vi "Standard ABR.vi"(11 "State (in)":T17) -> (3 "State":T17)   [LabVIEW 2020]
uses:
  epl-vi-lib/Utility VIs/Buttons/KCheckmarkBoolean 2.ctl
  CFTS VIs/CFTS-Experiment State.ctl
  Typedefs/ABR-Analysis State.ctl
  Threshold Estimation VIs/ABR3-Threshold Estimation Result.ctl
  <vilib>/printing/EasyPrintingControls.llb/layout_options.ctl
  <vilib>/printing/EasyPrintingControls.llb/orientation.ctl
  <vilib>/printing/EasyPrintingControls.llb/panel_scaling_for_page.ctl
  <vilib>/printing/EasyPrintingControls.llb/margins.ctl
  <vilib>/printing/EasyPrintingControls.llb/margin_values.ctl
  <vilib>/printing/EasyPrintingControls.llb/measurement_system.ctl
  <vilib>/printing/EasyPrintingControls.llb/printer_options.ctl
  <vilib>/printing/EasyPrintingControls.llb/printing_method.ctl
  <vilib>/printing/EasyPrintingControls.llb/color_or_monochrome.ctl
  <vilib>/printing/EasyPrintingControls.llb/page_header_options.ctl
  <vilib>/printing/EasyPrintingControls.llb/page_headers.ctl
  <vilib>/printing/EasyPrintingControls.llb/page_header_content_options.ctl
  Typedefs/ABR-Queue Data.ctl
  Typedefs/ABR-Parameters.ctl
  Typedefs/ABR-Stimulus.ctl
  Typedefs/ABR-Sequence.ctl
  Typedefs/ABR-Response.ctl
  Threshold Estimation VIs/ABR3-Threshold Estimation Parameters.ctl
  CFTS VIs/CFTS-Options.ctl
  <vilib>/printing/EasyPrintingControls.llb/contents.ctl
  f492785b-1e3c-4081-aebf-1185a71f0bc8.vi
  epl-vi-lib/Utility VIs/File IO VIs/Read Write Anything/Read Anything.vi
  <vilib>/printing/EasyPrinting.llb/Easy Print VI Panel or Documentation (refnum).vi
  epl-vi-lib/Utility VIs/File IO VIs/Configuration File Wrapper VIs/Config-Write Key (string).vi
  <vilib>/Utility/NIReport.llb/NI_ReportGenerationCore.lvlib
panel:
  out "result":T1
  out "Thr":string caption="Threshold (dB SPL)"
  in  "layout options":T2={"orientation (unchanged)"=0, "panel scaling for page (unchanged)"=0, "margins"={"override VI margins (false)"=FALSE, "margins (1.00)"={"top"=1.0, "left"=1.0, "right"=1.0, "bottom"=1.0}, "measurement system (default)"=0}, "printer options"={"destination printer name (current)"="", "printing method (unchanged)"=0, "color or monochrome (unchanged)"=0}, "page header options"={"page headers (unchanged)"=0, "page header content options"={"Include VI Name"=TRUE, "Include VI Path"=TRUE, "Include Last Modification Date"=TRUE, "Include Date Printed"=TRUE, "Include Page Number"=TRUE, "Include VI Icon"=TRUE}}} {"page header options"."page headers (unchanged)" items=["Unchanged", "Include page headers", "Do not include page headers"]; "printer options"."color or monochrome (unchanged)" items=["Unchanged", "Color/grayscale", "Monochrome"]; "printer options"."printing method (unchanged)" items=["Unchanged", "Standard", "PostScript", "Bitmap"]; "panel scaling for page (unchanged)" items=["Unchanged", "No Scaling", "Scale front panel to fit"]; "orientation (unchanged)" items=["Unchanged", "portrait", "landscape"]; "margins"."measurement system (default)" items=["Default", "US", "Metric"]; "margins"."margins (1.00)"."right" format="%.2f"; "margins"."margins (1.00)"."bottom" format="%.2f"; "margins"."margins (1.00)"."top" format="%.2f"; "margins"."margins (1.00)"."left" format="%.2f"}
  out "CM":cluster{dbl[], dbl[]}[](graph) caption="\"CM\""
  out "Neural":cluster{dbl[], dbl[]}[](graph)
  in  "NOTES":string
  out "Analysis":T14
  in  "Response":T16={"Gain"=10000, "Averages"=512, "Window (ms)"=8.5, "Thr Fast Steps"=1.5} {"Thr Fast Steps" format="%.2f"; "Window (ms)" format="%.2f"}
  in  "CAP or ABR":enum16{"CAP", "ABR"}(ring)=enum."ABR" caption="Measure what"
  out "MAX SPL":dbl=113.05999755859375 format="%.2f"
  out "SPL":dbl=35.0
  out "User":string
  out "Run #":u16=14
  out "ID #":u16=1
  in  "Stimulus":T18={"Destination"=1, "Waveform"=enum."TONE PIP", "Frequency (kHz)"=16.0, "Rep rate (/sec)"=30.0, "Alternate Polarity"=FALSE, "Start (dB)"=20, "Stop (dB)"=80, "Step (dB)"=5} {"Rep rate (/sec)" format="%#_8g"; "Frequency (kHz)" format="%.2f"; "Start (dB)" step=5; "Destination" items=["Right ear", "Left ear", "Speaker"]}
  in  "Norm":T19=TRUE caption="Normalize individual traces"
  out "CLICK I-O":cluster{dbl[], dbl[]}[](graph)
  in  "START":bool
  in  "RETURN":bool
  in  "STOP":bool
  out "TONE I-O":cluster{dbl[], dbl[]}[](graph)
  # "Response"
  # "Running Average"
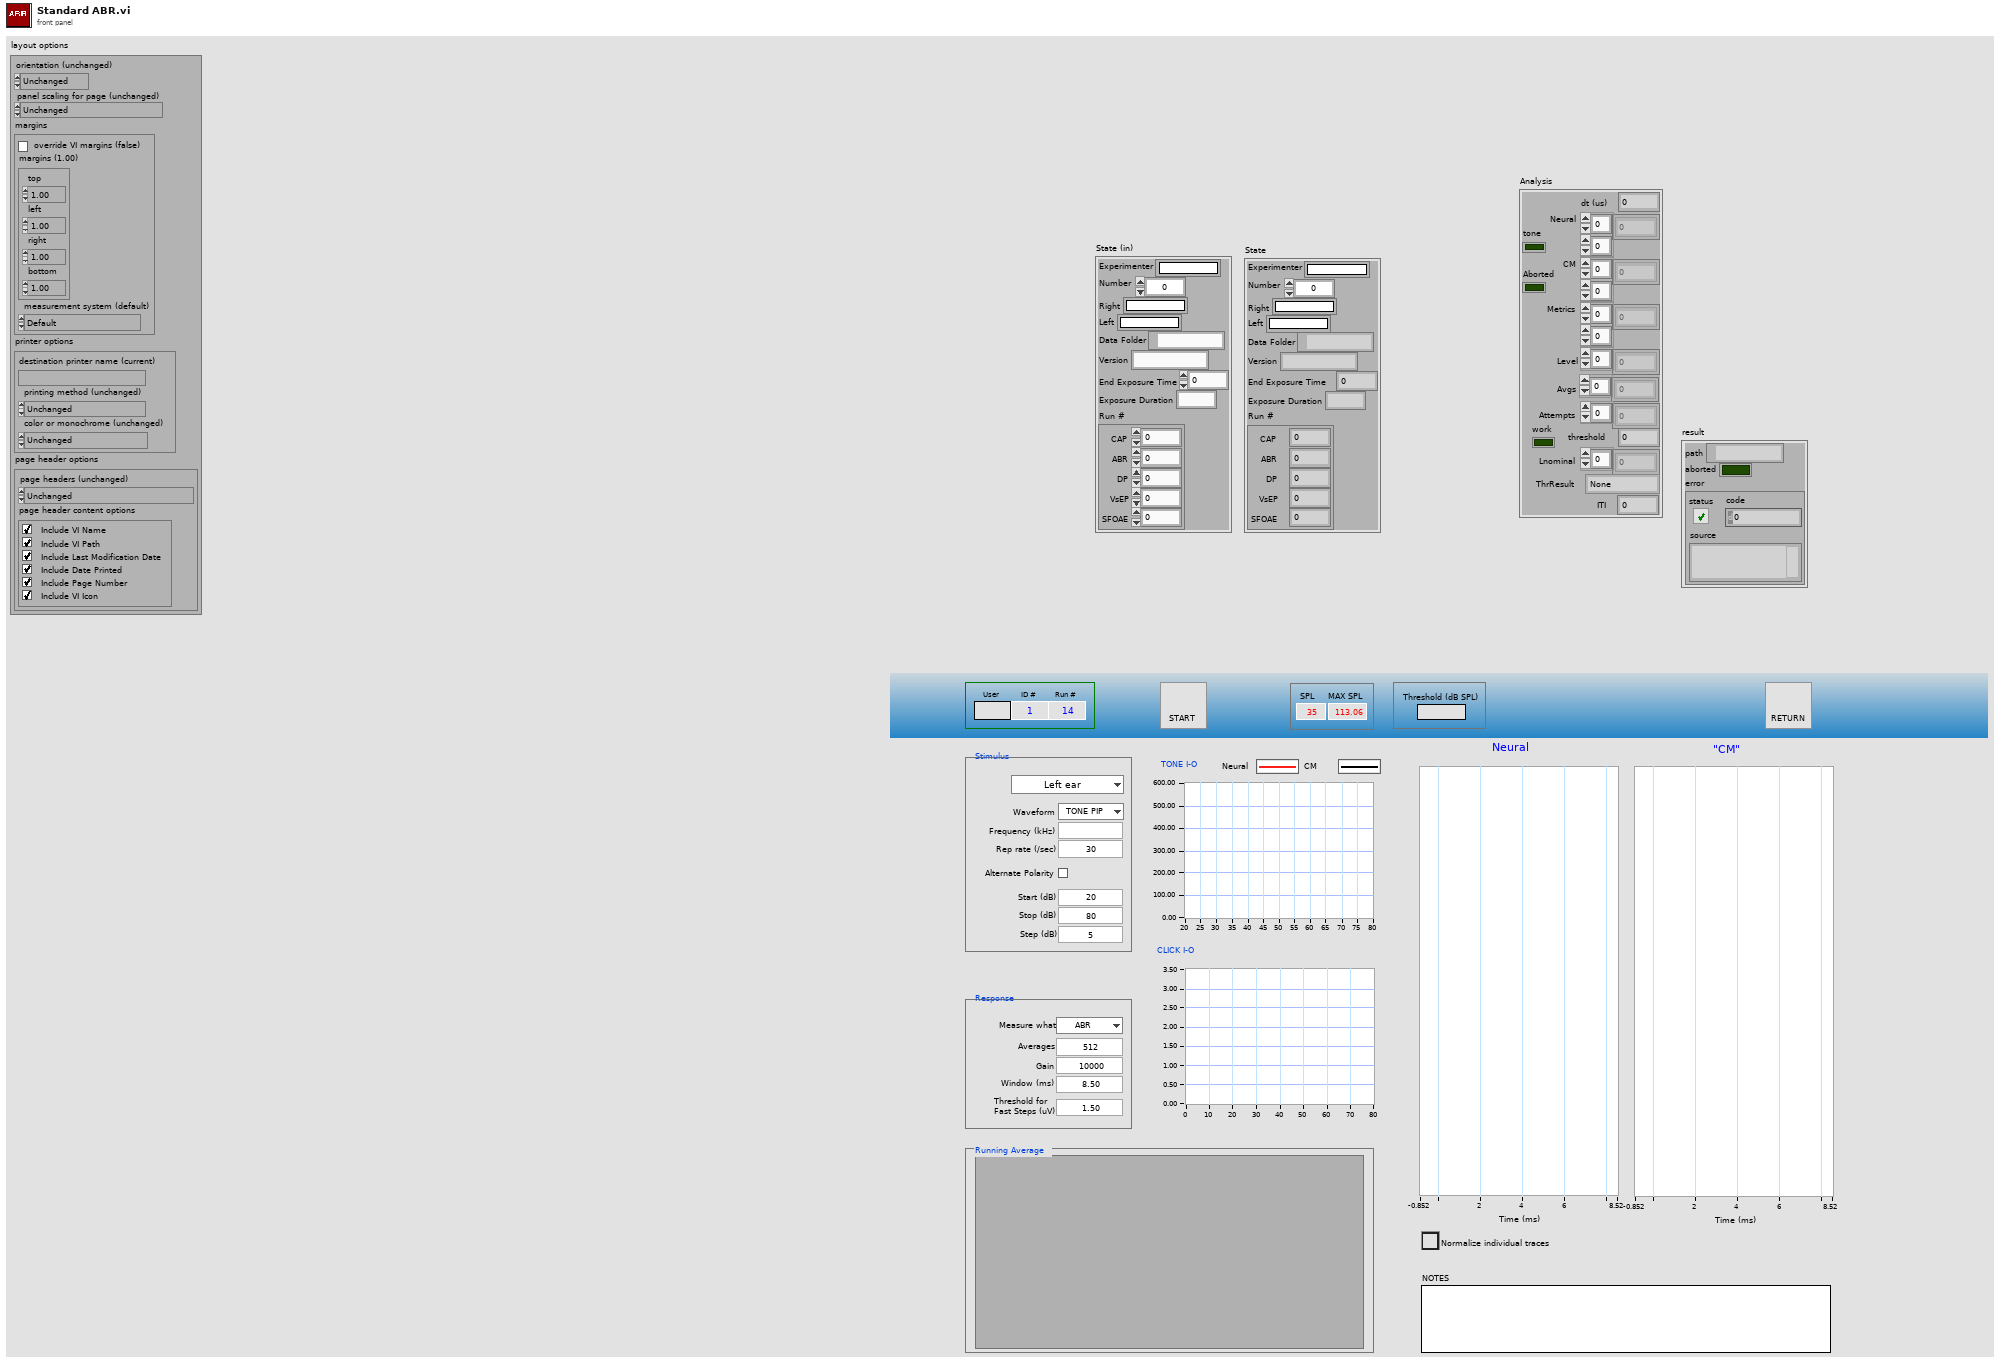
[diagram p1: front panel]
types:
  T1 = cluster{"path":path, "aborted":bool, "error":errorcluster}
  T2 = typedef "NI_ReportGenerationCore.lvlib/layout_options.ctl" = cluster{"orientation (unchanged)":T3, "panel scaling for page (unchanged)":T4, "margins":T5, "printer options":T8, "page header options":T11}
  T3 = typedef "NI_ReportGenerationCore.lvlib/orientation.ctl" = u16
  T4 = typedef "NI_ReportGenerationCore.lvlib/panel_scaling_for_page.ctl" = u16
  T5 = typedef "NI_ReportGenerationCore.lvlib/margins.ctl" = cluster{"override VI margins (false)":bool, "margins (1.00)":T6, "measurement system (default)":T7}
  T6 = typedef "NI_ReportGenerationCore.lvlib/margin_values.ctl" = cluster{"top":dbl, "left":dbl, "right":dbl, "bottom":dbl}
  T7 = typedef "NI_ReportGenerationCore.lvlib/measurement_system.ctl" = u16
  T8 = typedef "NI_ReportGenerationCore.lvlib/printer_options.ctl" = cluster{"destination printer name (current)":string, "printing method (unchanged)":T9, "color or monochrome (unchanged)":T10}
  T9 = typedef "NI_ReportGenerationCore.lvlib/printing_method.ctl" = u16
  T10 = typedef "NI_ReportGenerationCore.lvlib/color_or_monochrome.ctl" = u16
  T11 = typedef "NI_ReportGenerationCore.lvlib/page_header_options.ctl" = cluster{"page headers (unchanged)":T12, "page header content options":T13}
  T12 = typedef "NI_ReportGenerationCore.lvlib/page_headers.ctl" = u16
  T13 = typedef "NI_ReportGenerationCore.lvlib/page_header_content_options.ctl" = cluster{"Include VI Name":bool, "Include VI Path":bool, "Include Last Modification Date":bool, "Include Date Printed":bool, "Include Page Number":bool, "Include VI Icon":bool}
  T14 = typedef "ABR-Analysis State.ctl" = cluster{"dt (us)":dbl, "Neural":dbl[][], "CM":dbl[][], "Metrics":dbl[][], "Level":dbl[], "Avgs":i32[], "Attempts":i32[], "Aborted":bool, "threshold":dbl, "Lnominal":dbl[], "tone":bool, "work":bool, "ThrResult":T15, "ITI":dbl}
  T15 = typedef "ABR3-Threshold Estimation Result.ctl" = enum16{"None", "Power", "Sigmoid", "Power (noisy)", "Suprathreshold", "Invalid"}
  T16 = cluster{"Gain":i32, "Averages":i32, "Window (ms)":sgl, "Thr Fast Steps":sgl}
  T17 = typedef "CFTS-Experiment State.ctl" = cluster{"Experimenter":string, "Number":u32, "Right":string, "Left":string, "Data Folder":path, "Version":string, "End Exposure Time":dbl, "Exposure Duration":string, "Run #":cluster{"CAP":i32, "ABR":i32, "DP":i32, "VsEP":i32, "SFOAE":i32}}
  T18 = cluster{"Destination":u16, "Waveform":enum16{"TONE PIP", "CLICK"}, "Frequency (kHz)":ext, "Rep rate (/sec)":dbl, "Alternate Polarity":bool, "Start (dB)":i32, "Stop (dB)":i32, "Step (dB)":i32}
  T19 = typedef "KCheckmarkBoolean 2.ctl" = bool
  T20 = typedef "ABR-Queue Data.ctl" = cluster{"action":string, "Path":path, "Params":T21, "Threshold Estimation":T25}
  T21 = typedef "ABR-Parameters.ctl" = cluster{"Stimulus":T22, "Sequence":T23, "Response":T24, "Normalize":bool, "Reject":dbl}
  T22 = typedef "ABR-Stimulus.ctl" = cluster{"Destination":string, "Waveform":enum16{"TONE PIP", "CLICK"}, "Frequency (kHz)":ext, "Rep rate (/sec)":dbl, "Alternate Polarity":bool, "Sampling rate (Hz)":dbl, "Duration (ms)":dbl, "Ramp (ms)":dbl, "Click width (us)":dbl, "ITI":enum16{"Rate", "Interval"}}
  T23 = typedef "ABR-Sequence.ctl" = cluster{"Start (dB)":i32, "Stop (dB)":i32, "Step (dB)":i32}
  T24 = typedef "ABR-Response.ctl" = cluster{"CAP or ABR":enum16{"CAP", "ABR"}, "Gain":i32, "Averages":i32, "Window (ms)":sgl, "Thr Fast Steps":sgl, "Fs (Hz)":dbl, "Save raw":bool}
  T25 = typedef "ABR3-Threshold Estimation Parameters.ctl" = cluster{"Tmin (ms)":dbl, "Tmax (ms)":dbl, "CC criterion":dbl, "adjR2 criterion":dbl}
  T26 = cluster{"TONE I-O":refnum<vi>, "Neural":refnum<vi>, "CM":refnum<vi>, "CLICK I-O":refnum<vi>}
  T27 = typedef "ABR-Runtime Data.ctl" = cluster{"Ceiling":dbl, "Threshold":dbl, "Crossed?":bool, "Step":dbl, "Stop":i32, "Avgs":i32, "Level":dbl, "AI Npts":i32, "Doubled?":bool, "dt":dbl, "gain":dbl, "rep pairs/buffer":i32, "NWinPts":i32, "Save raw":bool, "SigMan":refnum<class "SignalManager.lvclass">, "path":path}
  T28 = typedef "ABR-Averaging Result.ctl" = cluster{"navg":i32, "natt":i32, "Neural":dbl[], "Microphonic":dbl[]}
  T29 = cluster{"Datafile path":path, "abort":bool, "error out":errorcluster}
  T30 = typedef "CFTS-Options.ctl" = cluster{"Rig ID":string, "Acoustic System IDs":cluster{"Right":string, "Left":string}, "Extension":string, "Advanced users":string[], "All advanced":bool, "Run vitals":bool, "hash":string, "Allow nonEPL":bool, "NonEPL":string[], "Data root":path}
  T31 = enum8{"Enabled", "Disabled", "Disabled and Grayed Out"}
  T32 = cluster{string, "appended path":path, "Params":T21, "Threshold Estimation":T25}
  T33 = typedef "NI_ReportGenerationCore.lvlib/contents.ctl" = u16
  T34 = typedef "ABR3-Threshold Estimation Work.ctl" = cluster{"Threshold":dbl, "Criterion":dbl, "graphs":cluster{"X":dbl[], "Y":dbl[]}[], "Power2":string, "Sigmoid":string, "Result":T15}
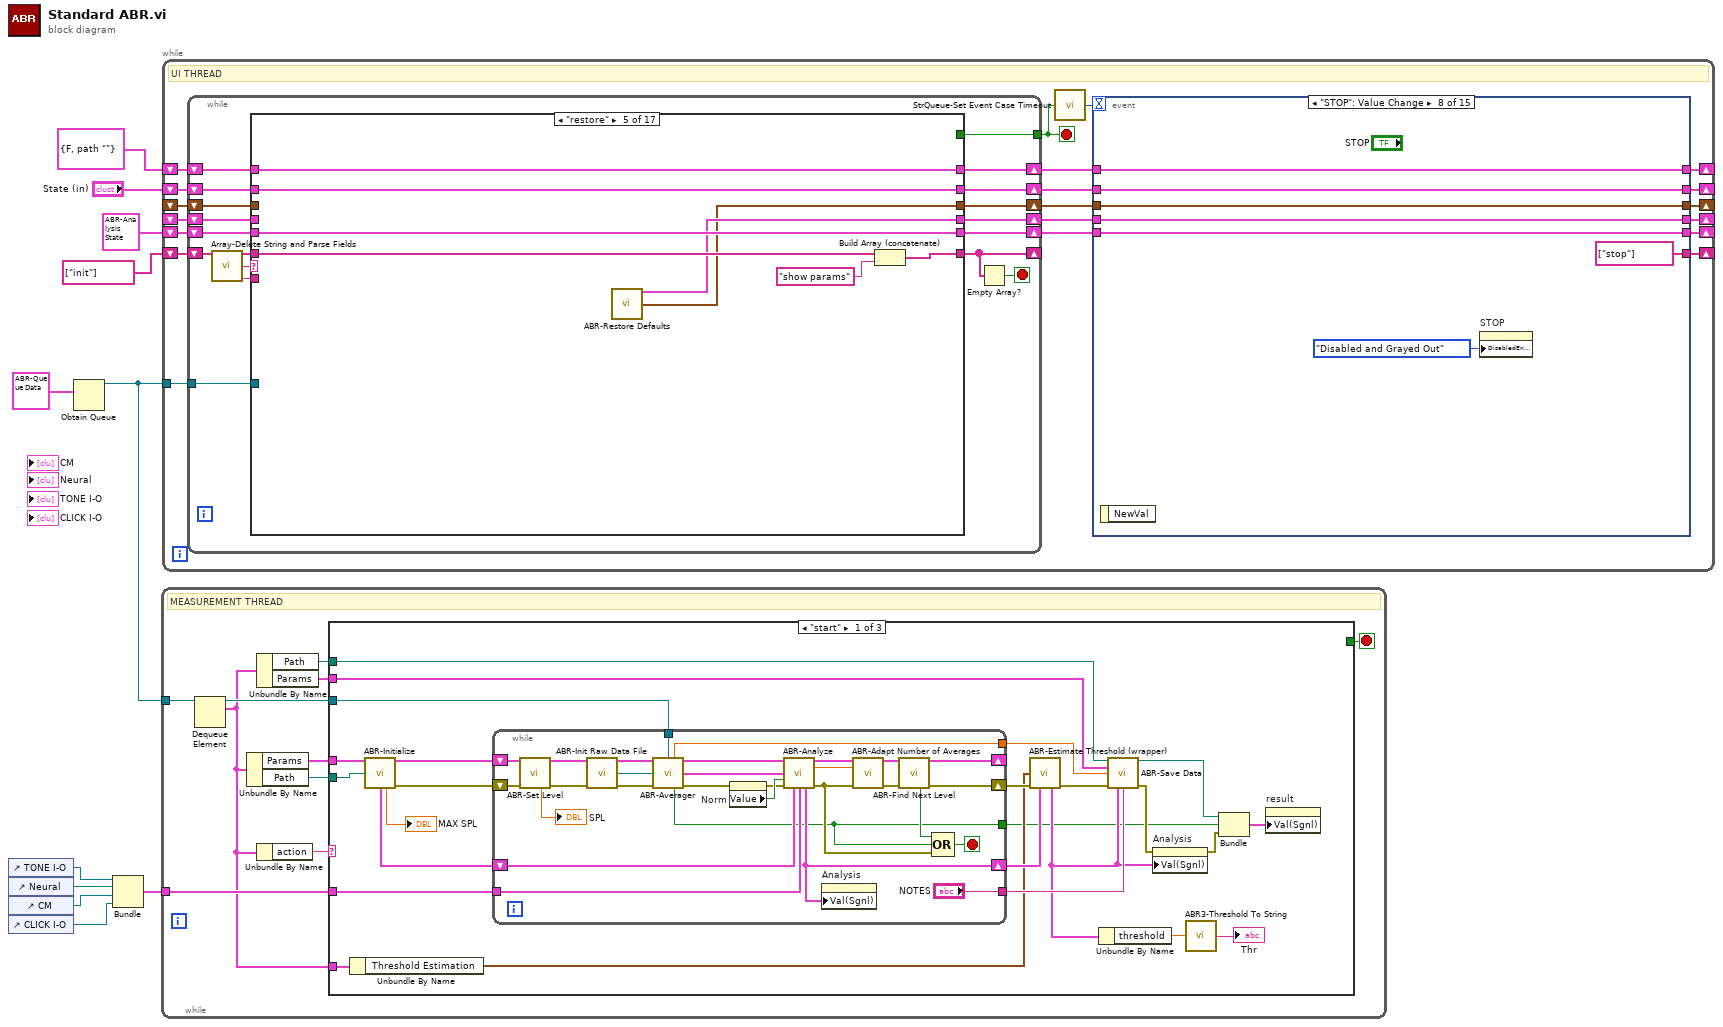
[diagram p0: block diagram]
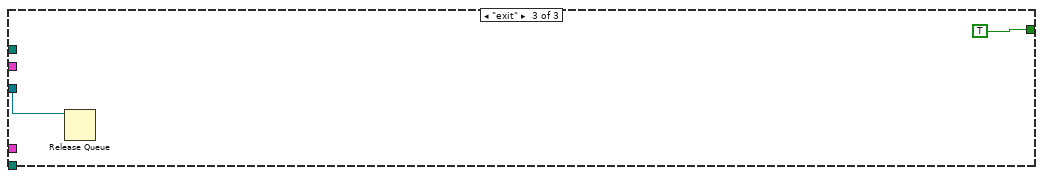
[diagram p3: hidden frame]
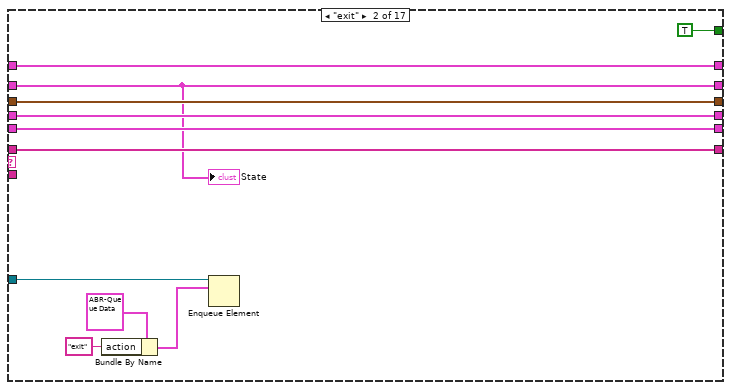
[diagram p5: hidden frame]
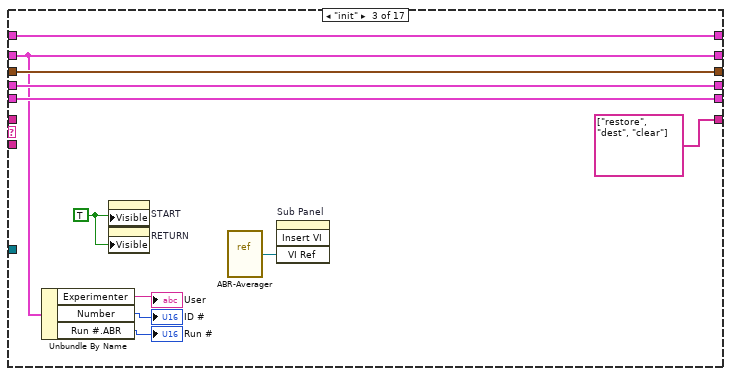
[diagram p6: hidden frame]
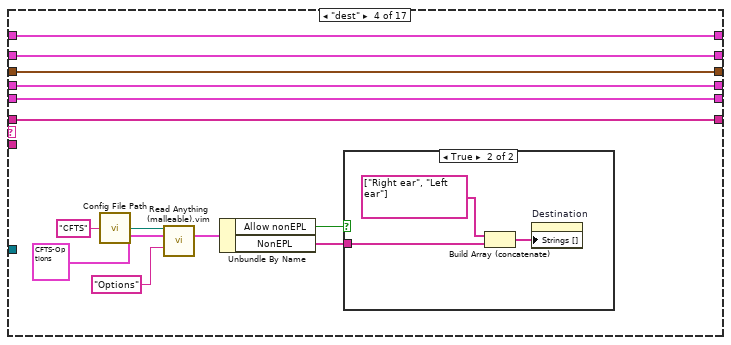
[diagram p7: hidden frame]
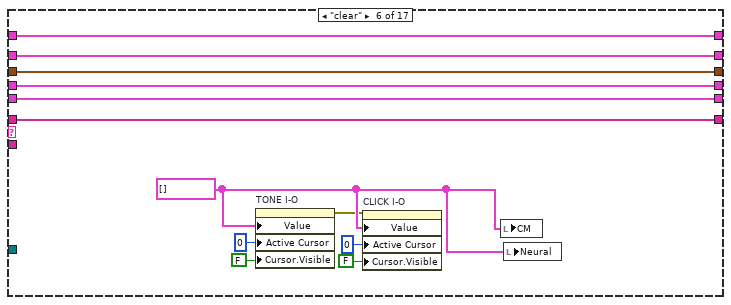
[diagram p9: hidden frame]
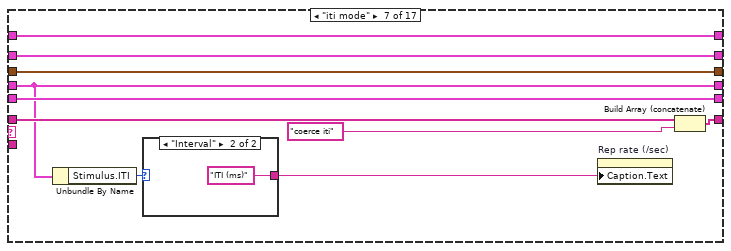
[diagram p10: hidden frame]
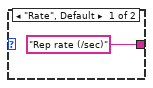
[diagram p11: hidden frame]
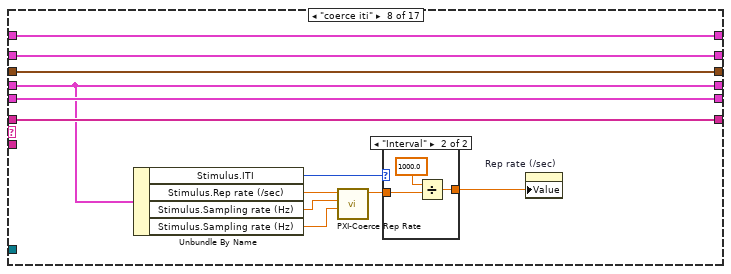
[diagram p12: hidden frame]
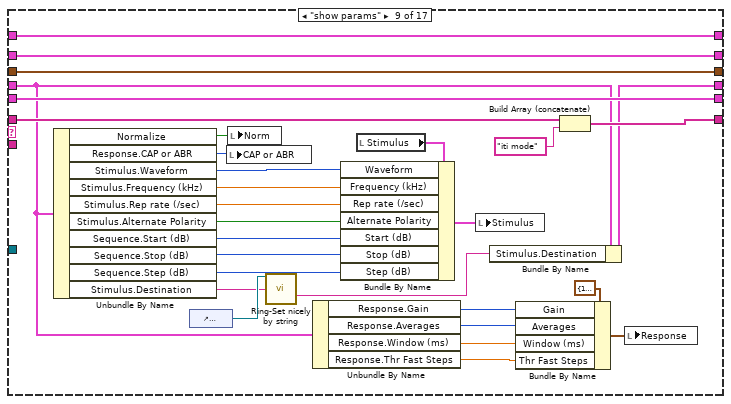
[diagram p14: hidden frame]
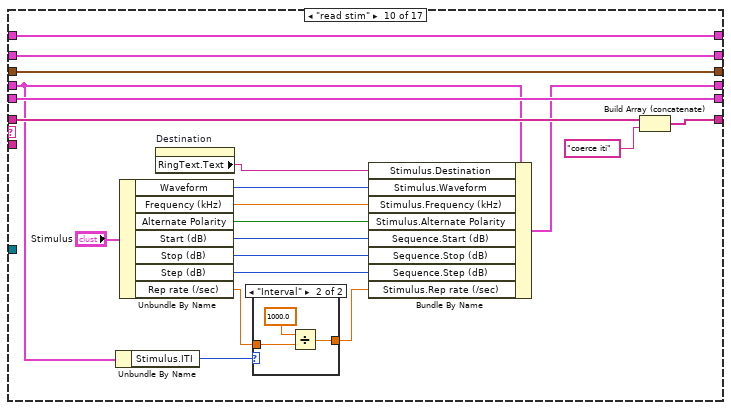
[diagram p15: hidden frame]
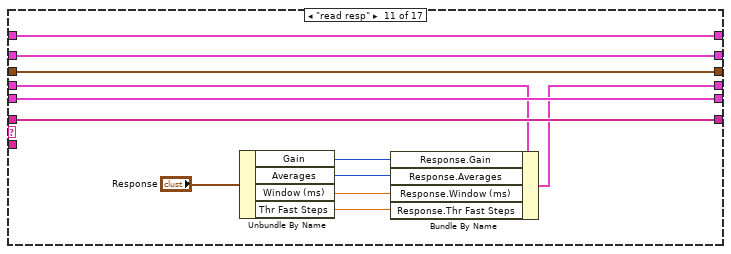
[diagram p17: hidden frame]
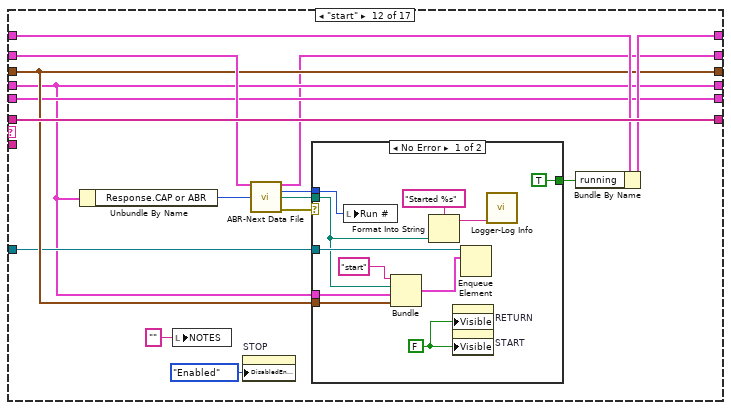
[diagram p18: hidden frame]
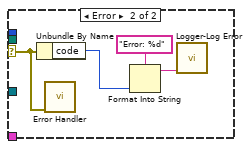
[diagram p19: hidden frame]
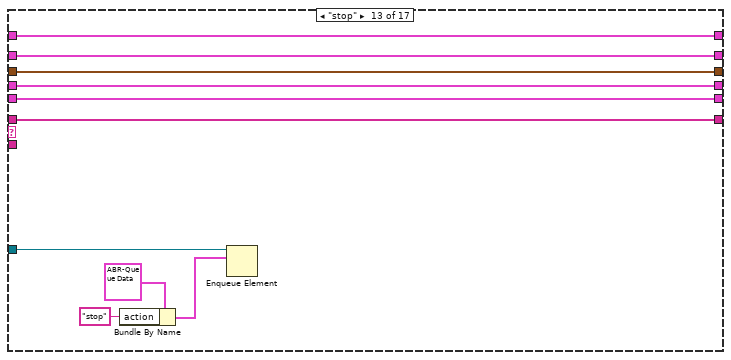
[diagram p20: hidden frame]
diagram:
  n1 = control-ref of="TONE I-O"() -> (w5:refnum<vi>)
  n2 = control-ref of="Neural"() -> (w7:refnum<vi>)
  n3 = control-ref of="CM"() -> (w6:refnum<vi>)
  n4 = control-ref of="CLICK I-O"() -> (w4:refnum<vi>)
  n5 = Obtain Queue(element data type=T20 {"action"="", "Path"=path "", "Params"={"Stimulus"={"Destination"="", "Waveform"=enum."TONE PIP", "Frequency (kHz)"=16.0, "Rep rate (/sec)"=30.0, "Alternate Polarity"=FALSE, "Sampling rate (Hz)"=0.0, "Duration (ms)"=30.0, "Ramp (ms)"=5.0, "Click width (us)"=0.0, "ITI"=enum."Rate"}, "Sequence"={"Start (dB)"=20, "Stop (dB)"=80, "Step (dB)"=5}, "Response"={"CAP or ABR"=enum."ABR", "Gain"=10000, "Averages"=512, "Window (ms)"=8.5, "Thr Fast Steps"=8.5, "Fs (Hz)"=25000.0, "Save raw"=FALSE}, "Normalize"=FALSE, "Reject"=0.0}, "Threshold Estimation"={"Tmin (ms)"=0.0, "Tmax (ms)"=0.0, "CC criterion"=0.0, "adjR2 criterion"=0.0}} ("Cluster")) -> (queue out=w11:refnum<queue>)  [unwired: 4 in, 2 out]
  n6 = Bundle("TONE I-O"=w5, "Neural"=w7, "CM"=w6, "CLICK I-O"=w4) -> (w8:T26)  [unwired: 1 in]
  n7 = while {
    tunnel: w11 -> [w21]
    tunnel: w8 -> [w20]
    stop <- w17 stop-if-true
    # "MEASUREMENT THREAD"
    n8 = Dequeue Element(queue=w21) -> (queue out=w19:refnum<queue>, element=w14:T20)  [unwired: 2 in, 2 out]
    n9 = Unbundle By Name(w14) -> ("Params"=w16:T21, "Path"=w15:path)
    n10 = Unbundle By Name(w14) -> ("Path"=w13:path, "Params"=w12:T21)
    n11 = Unbundle By Name(w14) -> ("action"=w18:string)
    n12 = case shown="\"start\"" w18 {
      tunnel: w20 -> [w46 _ _]
      tunnel: w19 -> [w36 _ w77]
      tunnel: [_ _ TRUE] -> w17
      tunnel: w16 -> [w44 _ _]
      tunnel: w15 -> [w40 _ _]
      tunnel: w14 -> [w31 _ _]
      tunnel: w13 -> [w28 _ _]
      tunnel: w12 -> [w27 _ _]
      frame "start" {
        n13 = Unbundle By Name(w31) -> ("Threshold Estimation"=w30:T25)
        n14 = call "ABR-Initialize.vi"("Params"=w44, "Data path"=w40) -> ("Runtime"=w41:T27, "Analysis"=w42:T14, "Ceiling"=→"MAX SPL":dbl, "error out"=w43:errorcluster)  [unwired: 10 in]
        n15 = while {
          shift-right: [w74] -> w38
          shift-left: w43 -> [w72]
          shift-right: [w70] -> _
          shift-left: w41 -> [w69]
          shift-right: [w60] -> w37
          shift-left: w42 -> [w65]
          tunnel: w46 -> [w64]
          tunnel: ["NOTES"] -> w39
          tunnel: [w51] -> w26
          tunnel: w36 -> [w50]
          tunnel: [w47] -> w22
          stop <- w75 stop-if-true
          # "stepsize"
          # "max SPL"
          # "array of levels"
          # "current SPL"
          n16 = call "ABR-Set Level.vi"("Runtime"=w69, "error in (no error)"=w72) -> ("Runtime thru"=w59:T27, "Level"=→"SPL":dbl, "error out"=w57:errorcluster)  [unwired: 11 in]
          n17 = call "ABR-Init Raw Data File.vi"("Runtime in"=w59, "error in (no error)"=w57) -> ("Runtime out"=w58:T27, "refnum out"=w55:refnum<file>, "error out"=w56:errorcluster)  [unwired: 11 in]
          n18 = call "ABR-Averager.vi"("Runtime"=w58, "queue"=w50, "raw data file"=w55, "error in (no error)"=w56) -> ("Rej Thresh out"=w47:dbl, "Runtime thru"=w54:T27, "result"=w49:T28, "abort"=w51:bool, "error out"=w68:errorcluster)  [unwired: 7 in]
          n19 = property on="Norm" class="Bool (strict)"(error in=w68) -> (error out=w66:errorcluster, "Value"=w67:T19)  [unwired: 1 in, 1 out]
          n20 = call "ABR-Analyze.vi"("Runtime"=w54, "result"=w49, "Normalize individual?"=w67, "error in"=w66, "Analysis in"=w65, "Graphs"=w64) -> ("Runtime thru"=w53:T27, "spread value"=w48:dbl, "Analysis out"=w60:T14, "error out"=w52:errorcluster)  [unwired: 6 in]
          n21 = property on="Analysis" class="Clust (strict)"("Val(Sgnl)"=w60) -> ()  [unwired: 2 in, 2 out]
          n22 = call "ABR-Adapt Number of Averages.vi"("Runtime"=w53, "Amplitude"=w48, "error in (no error)"=w52) -> ("Runtime out"=w63:T27, "error out"=w62:errorcluster)  [unwired: 11 in]
          n23 = call "ABR-Find Next Level.vi"("Runtime"=w63, "error in (no error)"=w62) -> ("Runtime out"=w70:T27, "Finished"=w73:bool, "error out"=w74:errorcluster)  [unwired: 11 in]
          n24 = Compound Arithmetic op=OR(w73, w51, w52) -> (w75:bool)
        }
        n25 = call "ABR-Estimate Threshold (wrapper).vi"("Threshold Estimation"=w30, "error in (no error)"=w38, "Analysis (in)"=w37) -> ("Analysis (out)"=w32:T14, "error out"=w35:errorcluster)  [unwired: 10 in, 1 out]
        n26 = Unbundle By Name(w32) -> ("threshold"=w33:dbl)
        n27 = call "ABR-Save Data.vi"("file path"=w28, "Params"=w27, "reject"=w22, "error in (no error)"=w35, "Analysis"=w32, "Notes"=w39) -> ("Datafile path"=w24:path, "error out"=w29:errorcluster)  [unwired: 8 in]
        n28 = property on="Analysis" class="Clust (strict)"(error in=w29, "Val(Sgnl)"=w32) -> (error out=w25:errorcluster)  [unwired: 1 in, 1 out]
        n29 = call "ABR3-Threshold To String.vi"("Threshold"=w33) -> ("String"=→"Thr":string)
        n30 = Bundle("Datafile path"=w24, "abort"=w26, "error out"=w25) -> (w23:T29)  [unwired: 1 in]
        n31 = property on="result" class="Clust (strict)"("Val(Sgnl)"=w23) -> ()  [unwired: 2 in, 2 out]
      }
      frame "stop", Default {
      }
      frame "exit" {
        n32 = Release Queue(queue=w77) -> ()  [unwired: 2 in, 3 out]
      }
    }
  }
  n33 = while {
    tunnel: w11 -> [w83]
    shift-right: [w90] -> _
    shift-left: _ -> [w88]
    shift-right: [w91] -> _
    shift-left: T14 {"dt (us)"=0.0, "Neural"=[], "CM"=[], "Metrics"=[], "Level"=[], "Avgs"=[], "Attempts"=[], "Aborted"=FALSE, "threshold"=0.0, "Lnominal"=[], "tone"=FALSE, "work"=FALSE, "ThrResult"=enum."None", "ITI"=0.0} ("Analysis") -> [w92]
    shift-right: [w89] -> _
    shift-left: _ -> [w86]
    shift-right: [w96] -> _
    shift-left: string[] ["init"] -> [w97]
    shift-right: [w80] -> _
    shift-left: cluster{"running":bool, "path":path} {"running"=FALSE, "path"=path ""} -> [w82]
    shift-right: [w79] -> _
    shift-left: "State (in)" -> [w84]
    stop <- w94 stop-if-true
    # "UI THREAD"
    n34 = while {
      shift-right: [w114] -> _
      shift-left: w97 -> [w100]
      tunnel: [w112] -> w94
      shift-right: [w109] -> w85
      shift-left: w88 -> [w108]
      shift-right: [w111] -> w93
      shift-left: w92 -> [w110]
      shift-right: [w107] -> w87
      shift-left: w86 -> [w106]
      tunnel: w83 -> [w104]
      shift-right: [w102] -> w81
      shift-left: w82 -> [w103]
      shift-right: [w101] -> w78
      shift-left: w84 -> [w105]
      stop <- w113 stop-if-true
      n35 = call "Array-Delete String and Parse Fields.vi"("Array in"=w100) -> ("Array out"=w115:string[], "Field 1"=w99:string, "Field 2"=w98:string)  [unwired: 10 in, 2 out]
      n36 = case shown="\"restore\"" w99 {
        tunnel: w115 -> [w121 w132 _ w156 w167 w179 w189 w203 w236 w256 w272 w288 w313 w323 w362 w378 w392]
        tunnel: [w121 w132 string[] ["restore", "dest", "clear"] w156 w161 w179 w187 w203 w235 w255 w272 w288 w313 w321 w362 w378 w392] -> w114
        tunnel: [_ TRUE _ _ _ _ _ _ _ _ _ _ _ _ _ _ _] -> w112
        tunnel: [w118 w130 w143 w155 w166 w178 w184 w201 w233 w253 w270 w282 w312 w328 w355 w363 w383] -> w111
        tunnel: w110 -> [w118 w130 w143 w155 w166 w178 w184 w201 w233 w253 w270 w282 w312 w328 w355 w363 w384]
        tunnel: [w119 w129 w142 w154 w165 w177 w183 w195 w212 w242 w261 w280 w311 w314 w361 w377 w391] -> w109
        tunnel: w108 -> [w119 w129 w142 w154 _ w177 w183 w195 w214 w240 w266 w280 w311 w314 w361 w377 w391]
        tunnel: [w120 w128 w141 w153 w164 w176 w185 w202 w234 w254 w271 w283 w310 w327 w360 w376 w385] -> w107
        tunnel: w106 -> [w120 w128 w141 w153 _ w176 w185 w202 w234 w254 w271 w283 w310 w327 w360 w376 w385]
        tunnel: w105 -> [w116 w122 w137 w151 w162 w168 w180 w199 w209 w244 w268 w284 w308 w318 w358 w374 w382]
        tunnel: w104 -> [_ w125 _ _ _ _ _ _ _ _ _ w281 w304 _ _ _ _]
        tunnel: w103 -> [w117 w123 w133 w152 w163 w169 w181 w200 w210 w245 w269 w287 w309 w317 w359 w375 w390]
        tunnel: [w117 w123 w133 w152 w163 w169 w181 w200 w210 w245 w269 w285 w309 w316 w359 w375 w390] -> w102
        tunnel: [w116 w122 w137 w151 w162 w168 w180 w199 w209 w244 w268 w273 w308 w315 w358 w374 w382] -> w101
        tunnel: w98 -> [_ _ _ _ _ _ _ _ _ _ _ _ _ w320 _ _ _]
        frame "", Default {
        }
        frame "exit" {
          n37 = Bundle By Name(cluster=T20 {"action"="", "Path"=path "", "Params"={"Stimulus"={"Destination"="", "Waveform"=enum."TONE PIP", "Frequency (kHz)"=16.0, "Rep rate (/sec)"=30.0, "Alternate Polarity"=FALSE, "Sampling rate (Hz)"=0.0, "Duration (ms)"=30.0, "Ramp (ms)"=5.0, "Click width (us)"=0.0, "ITI"=enum."Rate"}, "Sequence"={"Start (dB)"=20, "Stop (dB)"=80, "Step (dB)"=5}, "Response"={"CAP or ABR"=enum."ABR", "Gain"=10000, "Averages"=512, "Window (ms)"=8.5, "Thr Fast Steps"=8.5, "Fs (Hz)"=25000.0, "Save raw"=FALSE}, "Normalize"=FALSE, "Reject"=0.0}, "Threshold Estimation"={"Tmin (ms)"=0.0, "Tmax (ms)"=0.0, "CC criterion"=0.0, "adjR2 criterion"=0.0}} ("Cluster"), "action"="exit") -> (w124:T20)
          n38 = Enqueue Element(queue=w125, element=w124) -> ()  [unwired: 2 in, 3 out]
          "State" <- w122
        }
        frame "init" {
          w136 = TRUE
          n39 = Unbundle By Name(w137) -> ("Experimenter"=→"User":string, "Number"=→"ID #":u32, "Run #.ABR"=→"Run #":i32)
          n40 = property on="START" class="Bool"("Visible"=w136) -> ()  [unwired: 2 in, 2 out]
          n41 = property on="RETURN" class="Bool"("Visible"=w136) -> ()  [unwired: 2 in, 2 out]
          n42 = vi-ref "ABR-Averager.vi"() -> (w135:refnum<vi>)
          n43 = invoke on="Sub Panel" class="SubPanel" method="Insert VI"("VI Ref"=w135) -> ()  [unwired: 3 in, 4 out]
        }
        frame "dest" {
          n44 = call "Config File Path.vi"("AppName"="CFTS") -> ("Default config file name"=w149:path)
          n45 = call "Read Anything (malleable).vim"("Config file path"=w149, "Options in"=T30 {"Rig ID"="", "Acoustic System IDs"={"Right"="", "Left"=""}, "Extension"="", "Advanced users"=[], "All advanced"=FALSE, "Run vitals"=FALSE, "hash"="", "Allow nonEPL"=FALSE, "NonEPL"=[], "Data root"=path ""} ("Options"), "Section"="Options") -> ("Options out"=w146:T30)  [unwired: 9 in, 3 out]
          n46 = Unbundle By Name(w146) -> ("Allow nonEPL"=w145:bool, "NonEPL"=w144:string[])
          n47 = case shown="True" w145 {
            tunnel: w144 -> [_ w159]
            frame False {
            }
            frame True {
              n48 = Build Array (concatenate)(string[] ["Right ear", "Left ear"], w159) -> (w157:string[])
              n49 = property on="Destination" class="Ring (strict)"("Strings []"=w157) -> ()  [unwired: 2 in, 2 out]
            }
          }
        }
        frame "restore" {
          n50 = call "ABR-Restore Defaults.vi"() -> ("Params"=w165:T21, "Threshold Estimation"=w164:T25)  [unwired: 13 in, 1 out]
          n51 = Build Array (concatenate)(w167, "show params") -> (w161:string[])
        }
        frame "clear" {
          w175 = cluster{dbl[], dbl[]}[] [] ("TONE I-O")
          n52 = property on="TONE I-O" class="XYGraph (strict)"("Value"=w175, "Active Cursor"=u32 0, "Cursor.Visible"=FALSE) -> (error out=w172:errorcluster)  [unwired: 2 in, 1 out]
          n53 = property on="CLICK I-O" class="XYGraph (strict)"(error in=w172, "Value"=w175, "Active Cursor"=u32 0, "Cursor.Visible"=FALSE) -> ()  [unwired: 1 in, 2 out]
          n54 = local write "CM"(w175) -> ()
          n55 = local write "Neural"(w175) -> ()
        }
        frame "iti mode" {
          n56 = Unbundle By Name(w183) -> ("Stimulus.ITI"=w182:enum16{"Rate", "Interval"})
          n57 = case shown="\"Interval\"" w182 {
            tunnel: ["Rep rate (/sec)" ("Caption.Text") "ITI (ms)" ("Caption.Text")] -> w188
            frame "Rate", Default {
            }
            frame "Interval" {
            }
          }
          n58 = property on="Rep rate (/sec)" class="DigNum (strict)"("Caption.Text"=w188) -> ()  [unwired: 2 in, 2 out]
          n59 = Build Array (concatenate)(w189, "coerce iti") -> (w187:string[])
        }
        frame "coerce iti" {
          n60 = Unbundle By Name(w195) -> ("Stimulus.ITI"=w192:enum16{"Rate", "Interval"}, "Stimulus.Rep rate (/sec)"=w196:dbl, "Stimulus.Sampling rate (Hz)"=w194:dbl, "Stimulus.Sampling rate (Hz)"=w193:dbl)
          n61 = call "PXI-Coerce Rep Rate.vi"("AI sampling rate (Hz)"=w193, "AO sampling rate (Hz)"=w194, "Rep rate (Hz)"=w196) -> ("Coerced rep rate (Hz)"=w198:dbl)  [unwired: 5 in, 3 out]
          n62 = case shown="\"Interval\"" w192 {
            tunnel: w198 -> [w204 w207]
            tunnel: [w204 w206] -> w197
            frame "Rate", Default {
            }
            frame "Interval" {
              n63 = Divide(x=1000.0, y=w207) -> (x/y=w206:dbl)
            }
          }
          n64 = property on="Rep rate (/sec)" class="DigNum (strict)"("Value"=w197) -> ()  [unwired: 2 in, 2 out]
        }
        frame "show params" {
          n65 = Unbundle By Name(w214) -> ("Normalize"=w208:bool, "Response.CAP or ABR"=w232:enum16{"CAP", "ABR"}, "Stimulus.Waveform"=w230:enum16{"TONE PIP", "CLICK"}, "Stimulus.Frequency (kHz)"=w229:ext, "Stimulus.Rep rate (/sec)"=w228:dbl, "Stimulus.Alternate Polarity"=w227:bool, "Sequence.Start (dB)"=w226:i32, "Sequence.Stop (dB)"=w225:i32, "Sequence.Step (dB)"=w224:i32, "Stimulus.Destination"=w221:string)
          n66 = control-ref of="Destination"() -> (w222:refnum<vi>)
          n67 = local write "CAP or ABR"(w232) -> ()
          n68 = local write "Norm"(w208) -> ()
          n69 = call "Ring-Set nicely by string.vi"("Ring in"=w222, "Device"=w221) -> ("Selection"=w211:string)  [unwired: 9 in, 4 out]
          n70 = Unbundle By Name(w214) -> ("Response.Gain"=w220:i32, "Response.Averages"=w219:i32, "Response.Window (ms)"=w218:sgl, "Response.Thr Fast Steps"=w217:sgl)
          n71 = local read "Stimulus"() -> (w231:T18)
          n72 = Bundle By Name(cluster=w231, "Waveform"=w230, "Frequency (kHz)"=w229, "Rep rate (/sec)"=w228, "Alternate Polarity"=w227, "Start (dB)"=w226, "Stop (dB)"=w225, "Step (dB)"=w224) -> (w223:T18)
          n73 = local write "Stimulus"(w223) -> ()
          n74 = Bundle By Name(cluster=w214, "Stimulus.Destination"=w211) -> (w212:T21)
          n75 = Bundle By Name(cluster=T16 {"Gain"=10000, "Averages"=512, "Window (ms)"=8.5, "Thr Fast Steps"=1.5} ("Response"), "Gain"=w220, "Averages"=w219, "Window (ms)"=w218, "Thr Fast Steps"=w217) -> (w216:T16)
          n76 = Build Array (concatenate)(w236, "iti mode" ("String")) -> (w235:string[])
          n77 = local write "Response"(w216) -> ()
        }
        frame "read stim" {
          n78 = Unbundle By Name(w240) -> ("Stimulus.ITI"=w239:enum16{"Rate", "Interval"})
          n79 = Unbundle By Name("Stimulus") -> ("Waveform"=w252:enum16{"TONE PIP", "CLICK"}, "Frequency (kHz)"=w251:ext, "Alternate Polarity"=w250:bool, "Start (dB)"=w249:i32, "Stop (dB)"=w248:i32, "Step (dB)"=w247:i32, "Rep rate (/sec)"=w238:dbl)
          n80 = property on="Destination" class="Ring (strict)"() -> ("RingText.Text"=w241:string)  [unwired: 2 in, 2 out]
          n81 = case shown="\"Interval\"" w239 {
            tunnel: w238 -> [w257 w259]
            tunnel: [w257 w258] -> w237
            frame "Rate", Default {
            }
            frame "Interval" {
              n82 = Divide(x=1000.0, y=w259) -> (x/y=w258:dbl)
            }
          }
          n83 = Bundle By Name(cluster=w240, "Stimulus.Destination"=w241, "Stimulus.Waveform"=w252, "Stimulus.Frequency (kHz)"=w251, "Stimulus.Alternate Polarity"=w250, "Sequence.Start (dB)"=w249, "Sequence.Stop (dB)"=w248, "Sequence.Step (dB)"=w247, "Stimulus.Rep rate (/sec)"=w237) -> (w242:T21)
          n84 = Build Array (concatenate)(w256, "coerce iti" ("String")) -> (w255:string[])
        }
        frame "read resp" {
          n85 = Unbundle By Name("Response") -> ("Gain"=w265:i32, "Averages"=w264:i32, "Window (ms)"=w263:sgl, "Thr Fast Steps"=w262:sgl)
          n86 = Bundle By Name(cluster=w266, "Response.Gain"=w265, "Response.Averages"=w264, "Response.Window (ms)"=w263, "Response.Thr Fast Steps"=w262) -> (w261:T21)
        }
        frame "start" {
          n87 = Unbundle By Name(w280) -> ("Response.CAP or ABR"=w279:enum16{"CAP", "ABR"})
          n88 = local write "NOTES"("" ("NOTES")) -> ()
          n89 = property on="STOP" class="Bool"("DisabledEnum"=T31."Enabled" ("Disabled")) -> ()  [unwired: 2 in, 2 out]
          n90 = call "ABR-Next Data File.vi"("State in"=w284, "CAP or ABR"=w279) -> ("State out"=w273:T17, "Run"=w278:i32, "appended path"=w277:path, "error out"=w275:errorcluster)  [unwired: 10 in]
          n91 = case shown="No Error" w275 {
            selector: w275 -> [_ w303]
            tunnel: w283 -> [w299 _]
            tunnel: w281 -> [w296 _]
            tunnel: w280 -> [w295 _]
            tunnel: w278 -> [w294 _]
            tunnel: w277 -> [w290 _]
            tunnel: [TRUE _] -> w274
            frame No Error {
              w293 = FALSE ("ABI Abort")
              n92 = local write "Run #"(w294) -> ()
              n93 = Bundle("start", "appended path"=w290, "Params"=w295, "Threshold Estimation"=w299) -> (w297:T32)  [unwired: 1 in]
              n94 = Format Into String(format string="Started %s", w290) -> (resulting string=w289:string)  [unwired: 2 in, 1 out]
              n95 = property on="RETURN" class="Bool"("Visible"=w293) -> ()  [unwired: 2 in, 2 out]
              n96 = property on="START" class="Bool"("Visible"=w293) -> ()  [unwired: 2 in, 2 out]
              n97 = Enqueue Element(queue=w296, element=w297) -> ()  [unwired: 2 in, 3 out]
              n98 = call "Logger-Log Info.vi"("Message"=w289) -> ()  [unwired: 14 in, 1 out]
            }
            frame Error {
              n99 = Unbundle By Name(w303) -> ("code"=w301:i32)
              n100 = call "Error Handler.vi"("error in (no error)"=w303) -> ()  [unwired: 12 in, 3 out]
              n101 = Format Into String(format string="Error: %d", w301) -> (resulting string=w300:string)  [unwired: 2 in, 1 out]
              n102 = call "Logger-Log Error.vi"("Message"=w300) -> ()  [unwired: 14 in, 1 out]
            }
          }
          n103 = Bundle By Name(cluster=w287, "running"=w274) -> (w285:cluster{"running":bool, "path":path})
        }
        frame "stop" {
          n104 = Bundle By Name(cluster=T20 {"action"="", "Path"=path "", "Params"={"Stimulus"={"Destination"="", "Waveform"=enum."TONE PIP", "Frequency (kHz)"=16.0, "Rep rate (/sec)"=30.0, "Alternate Polarity"=FALSE, "Sampling rate (Hz)"=0.0, "Duration (ms)"=30.0, "Ramp (ms)"=5.0, "Click width (us)"=0.0, "ITI"=enum."Rate"}, "Sequence"={"Start (dB)"=20, "Stop (dB)"=80, "Step (dB)"=5}, "Response"={"CAP or ABR"=enum."ABR", "Gain"=10000, "Averages"=512, "Window (ms)"=8.5, "Thr Fast Steps"=8.5, "Fs (Hz)"=25000.0, "Save raw"=FALSE}, "Normalize"=FALSE, "Reject"=0.0}, "Threshold Estimation"={"Tmin (ms)"=0.0, "Tmax (ms)"=0.0, "CC criterion"=0.0, "adjR2 criterion"=0.0}} ("Cluster"), "action"="stop") -> (w305:T20)
          n105 = Enqueue Element(queue=w304, element=w305) -> ()  [unwired: 2 in, 3 out]
        }
        frame "dispose" {
          n106 = Unbundle By Name(w318) -> ("Data Folder"=w319:path)
          n107 = Two Button Dialog(message="Data collection was aborted.\nSave data?", 1:"No" ("F button name (\"Cancel\")"), 2:"Yes" ("T button name (\"OK\")")) -> (T button?=w322:bool)
          n108 = case shown="False" w322 {
            tunnel: w323 -> [_ w352]
            tunnel: [_ w352] -> w321
            tunnel: w320 -> [w341 _]
            tunnel: w319 -> [w342 _]
            tunnel: w318 -> [w333 w351]
            tunnel: w317 -> [w337 w353]
            tunnel: [w336 w353] -> w316
            tunnel: [w330 w351] -> w315
            tunnel: w314 -> [w334 _]
            frame False {
              n109 = Unbundle By Name(w334) -> ("Response.CAP or ABR"=w332:enum16{"CAP", "ABR"})
              n110 = Concatenate Strings(w341, ".*" ("string")) -> (w339:string)
              n111 = call "FileIO-Delete Files.vi"("Folder"=w342, "Pattern"=w339) -> ()  [unwired: 13 in, 1 out]
              n112 = Concatenate Strings("Deleted " ("string"), w339) -> (w329:string)
              n113 = case shown="\"CAP\"" w332 {
                tunnel: w333 -> [w345 w349]
                tunnel: [w343 w347] -> w331
                frame "ABR" {
                  n114 = Unbundle By Name(w345) -> ("Run #.ABR"=w346:i32)
                  n115 = Decrement(x=w346) -> (x-1=w344:i32)
                  n116 = Bundle By Name(cluster=w345, "Run #.ABR"=w344) -> (w343:T17)
                }
                frame "CAP" {
                  n117 = Unbundle By Name(w349) -> ("Run #.CAP"=w350:i32)
                  n118 = Decrement(x=w350) -> (x-1=w348:i32)
                  n119 = Bundle By Name(cluster=w349, "Run #.CAP"=w348) -> (w347:T17)
                }
              }
              n120 = call "Logger-Log Info.vi"("Message"=w329) -> ()  [unwired: 14 in, 1 out]
              n121 = call "CFTS-Write State.vi"("State"=w331) -> ("State thru"=w330:T17)  [unwired: 13 in, 1 out]
              n122 = Bundle By Name(cluster=w337, "path"=path "") -> (w336:cluster{"running":bool, "path":path})
            }
            frame True {
            }
          }
        }
        frame "replot" {
          n123 = control-ref of="Neural"() -> (w356:refnum<vi>)
          n124 = control-ref of="CM"() -> (w357:refnum<vi>)
          n125 = call "ABR-Plot Traces.vi"("Analysis"=w355, "Normalize individual?"="Norm", "Neural Ref"=w356, "CM Ref"=w357) -> ()  [unwired: 11 in, 1 out]
        }
        frame "plot thresh" {
          n126 = Unbundle By Name(w363) -> ("tone"=w364:bool)
          n127 = control-ref of="TONE I-O"() -> (w366:refnum<vi>)
          n128 = control-ref of="CLICK I-O"() -> (w367:refnum<vi>)
          n129 = control-ref of="Neural"() -> (w369:refnum<vi>)
          n130 = control-ref of="CM"() -> (w368:refnum<vi>)
          n131 = local read "Norm"() -> (w370:T19)
          n132 = Select(t=w366, s=w364, f=w367) -> (s? t:f=w365:refnum<vi>)
          n133 = call "ABR-Plot Metrics.vi"("Analysis"=w363, "I-O"=w365) -> ("error out"=w371:errorcluster)  [unwired: 13 in]
          n134 = Unbundle By Name(w363) -> ("ThrResult"=w372:T15)
          n135 = call "ABR-Plot Traces.vi"("Analysis"=w363, "Normalize individual?"=w370, "error in (no error)"=w371, "Neural Ref"=w369, "CM Ref"=w368) -> ("error out"=w373:errorcluster)  [unwired: 10 in]
          n136 = case shown="\"Power (noisy)\", \"Suprathreshold\"" w372 {
            selector: w372 -> [_ w380]
            tunnel: w373 -> [_ _]
            frame "None", Default {
            }
            frame "Power (noisy)", "Suprathreshold" {
              n137 = control-ref of="This VI"() -> (w379:refnum<vi>)
              n138 = call "ABR3-Threshold Warning Dialog.vi"("Result"=w380, "Parent VI"=w379) -> ()  [unwired: 14 in]
            }
          }
        }
        frame "open" {
          n139 = Unbundle By Name(w382) -> ("Data Folder"=w381:path)
          n140 = call "FileIO-Open Dialog.vi"("Default Folder"=w381, "pattern (all files)"="*") -> ("error out"=w387:errorcluster, "cancelled"=w388:bool, "selected path"=w389:path)  [unwired: 7 in]
          n141 = case shown="False" w388 {
            tunnel: w387 -> [w413 _]
            tunnel: w384 -> [_ w423]
            tunnel: [w396 w423] -> w383
            tunnel: w389 -> [w394 _]
            tunnel: w385 -> [w393 _]
            frame False {
              n142 = call "ABR-Read Data.vi"("Path"=w394, "error in (no error)"=w413) -> ("Analysis"=w399:T14, "error out"=w401:errorcluster)  [unwired: 10 in, 2 out]
              n143 = Unbundle By Name(w399) -> ("threshold"=w403:dbl, "tone"=w404:bool)
              n144 = control-ref of="TONE I-O"() -> (w406:refnum<vi>)
              n145 = control-ref of="CLICK I-O"() -> (w407:refnum<vi>)
              n146 = control-ref of="Neural"() -> (w410:refnum<vi>)
              n147 = control-ref of="CM"() -> (w409:refnum<vi>)
              n148 = Not A Number/Path/Refnum?(number/path/refnum=w403) -> (NaN/Path/Refnum?=w402:bool)
              n149 = local read "Norm"() -> (w411:T19)
              n150 = Select(t=w406, s=w404, f=w407) -> (s? t:f=w405:refnum<vi>)
              n151 = case shown="True" w402 {
                tunnel: w401 -> [w417 w422]
                tunnel: [w417 w421] -> w400
                tunnel: w399 -> [w416 w420]
                tunnel: [w416 w419] -> w396
                tunnel: w393 -> [_ w418]
                frame False {
                }
                frame True {
                  n152 = call "ABR-Estimate Threshold (wrapper).vi"("Threshold Estimation"=w418, "error in (no error)"=w422, "Analysis (in)"=w420) -> ("Analysis (out)"=w419:T14, "error out"=w421:errorcluster)  [unwired: 10 in, 1 out]
                }
              }
              n153 = Unbundle By Name(w396) -> ("threshold"=w398:dbl)
              n154 = call "ABR-Plot Metrics.vi"("Analysis"=w396, "error in (no error)"=w400, "I-O"=w405) -> ("error out"=w412:errorcluster)  [unwired: 12 in]
              n155 = call "ABR-Plot Traces.vi"("Analysis"=w396, "Normalize individual?"=w411, "error in (no error)"=w412, "Neural Ref"=w410, "CM Ref"=w409) -> ("error out"=w408:errorcluster)  [unwired: 10 in]
              n156 = call "ABR3-Threshold To String.vi"("Threshold"=w398) -> ("String"=w397:string)
              n157 = Unbundle By Name(w396) -> ("ThrResult"=w395:T15)
              n158 = call "Error Handler.vi"("error in (no error)"=w408) -> ()  [unwired: 12 in, 3 out]
              n159 = local write "Thr"(w397) -> ()
              n160 = case shown="\"Power (noisy)\", \"Suprathreshold\"" w395 {
                selector: w395 -> [_ w415]
                frame "None", Default {
                }
                frame "Power (noisy)", "Suprathreshold" {
                  n161 = control-ref of="This VI"() -> (w414:refnum<vi>)
                  n162 = call "ABR3-Threshold Warning Dialog.vi"("Result"=w415, "Parent VI"=w414) -> ()  [unwired: 14 in]
                }
              }
            }
            frame True {
            }
          }
        }
      }
      n163 = Empty Array?(array=w114) -> (empty?=w113:bool)
    }
    n164 = call "StrQueue-Set Event Case Timeout.vi"("Quit"=w94) -> ("timeout"=w95:i32)  [unwired: 14 in]
    n165 = event shown="[7] \"STOP\": Value Change" {
      selector: _ -> [_ _ _ _ _ _ _ _ _ _ _ _ _ _ _]
      dyn-events: _ -> [_ _ _ _ _ _ _ _ _ _ _ _ _ _ _]
      timeout: w95 -> [_ _ _ _ _ _ _ _ _ _ _ _ _ _ _]
      tunnel: w85 -> [w426 w435 w444 w498 w505 w511 w516 w524 w543 w562 w575 w590 w599 w605 w610]
      tunnel: [w426 w435 w443 w498 w505 w511 w516 w524 w543 w556 w575 w590 w598 w605 w610] -> w90
      tunnel: w93 -> [w428 w434 w438 w497 w504 w510 w517 w523 w541 w561 w574 w592 w596 w604 _]
      tunnel: [w428 w434 w442 w497 w503 w510 w517 w523 w541 w561 w574 w592 w596 w604 w609] -> w91
      tunnel: [w427 w432 w440 w494 w502 w509 w515 w522 w542 w560 w573 w591 w595 w603 w608] -> w89
      tunnel: w87 -> [w427 w432 w441 w494 w502 w509 w515 w522 w542 w560 w573 w591 w595 w603 w608]
      tunnel: [_ string[] ["exit"] w439 _ _ string[] ["exit"] string[] ["start"] string[] ["stop"] w533 string[] ["replot"] _ string[] ["read stim"] _ string[] ["read resp"] _] -> w96
      tunnel: w81 -> [w425 w430 w437 w493 w501 w507 w514 w521 w540 w559 w566 w588 w594 w602 w607]
      tunnel: [w425 w430 w437 w493 w501 w507 w514 w521 w527 w559 w566 w588 w594 w602 w607] -> w80
      tunnel: [w424 w429 w436 w492 w500 w506 w513 w520 w531 w558 w572 w587 w593 w601 w606] -> w79
      tunnel: w78 -> [w424 w429 w436 w492 w500 w506 w513 w520 w531 w558 w572 w587 w593 w601 w606]
      event Timeout {
        n166 = event-data() -> ()  [unwired: 1 in, 1 out]
      }
      event Panel Close? {
        n167 = event-data() -> ()  [unwired: 1 in, 1 out]
        n168 = event-data("Discard?"=TRUE) -> ()  [unwired: 1 in, 1 out]
      }
      event Menu Selection (User) {
        n169 = event-data() -> ("ItemTag"=w445:string)  [unwired: 1 in]
        n170 = case shown="\"mmEditOptions\"" w445 {
          tunnel: w444 -> [w448 w451 w460 w467 w474 w478 w480 w491]
          tunnel: [w448 w451 w460 w467 w474 w478 w479 w491] -> w443
          tunnel: w438 -> [w447 w452 w462 w466 w470 w477 w486 w489]
          tunnel: [w447 w452 w462 w466 w470 w477 w486 w489] -> w442
          tunnel: w441 -> [w446 w450 w454 w468 w469 w476 w485 w488]
          tunnel: [w446 w450 w454 w468 w469 w476 w484 w488] -> w440
          tunnel: [_ string[] ["restore"] _ string[] ["open"] _ string[] ["exit"] w482 _] -> w439
          frame "False", Default {
          }
          frame "mmFileRestore" {
          }
          frame "mmFileSave" {
            n171 = call "Config File Path.vi"("AppName"="CFTS") -> ("Default config file name"=w461:path)
            n172 = call "Write Anything.vi"("Section Name (Name of \"Anything\")"="Standard ABR" ("Section Name (Name of \"Anything\")"), "Anything"=w460, "Path (dialog)"=w461) -> ("Error Out"=w456:errorcluster, "Path out"=w457:path)  [unwired: 7 in]
            n173 = call "Write Anything.vi"("Error In"=w456, "Section Name (Name of \"Anything\")"="ABR Threshold" ("Section Name (Name of \"Anything\")"), "Anything"=w454, "Path (dialog)"=w457) -> ("Error Out"=w455:errorcluster)  [unwired: 6 in, 1 out]
            n174 = case shown="No Error" w455 {
              selector: w455 -> [_ w464]
              frame No Error {
                n175 = One Button Dialog(message="Defaults saved.") -> ()  [unwired: 1 in, 1 out]
              }
              frame Error {
                n176 = call "Error Handler.vi"("error in (no error)"=w464) -> ()  [unwired: 12 in, 3 out]
              }
            }
          }
          frame "mmFileOpen" {
          }
          frame "mmFilePrint" {
            w473 = T33 1 items=["Complete front panel", "Visible portion of front panel", "Icon, description, panel and diagram", "Documentation: Using the panel", "Documentation: Using as a subVI", "Documentation: Complete", "Documentation: Custom"] ("contents (complete front panel)")
            n177 = control-ref of="This VI"() -> (w471:refnum<vi>)
            n178 = call-poly <vilib>:"Easy Print VI Panel or Documentation.vi"("layout options"="layout options", "contents (complete front panel)"=w473, "VI reference"=w471) -> ()  [unwired: 7 in, 2 out]
          }
          frame "mmFileExit" {
          }
          frame "mmEditOptions" {
            n179 = control-ref of="This VI"() -> (w481:refnum<vi>)
            n180 = call "ABR-Options Dialog.vi"("Params in"=w480, "Parent VI"=w481, "Threshold Estimation In"=w485) -> ("Params out"=w479:T21, "Threshold Estimation Out"=w484:T25, "Canceled?"=w483:bool)  [unwired: 10 in]
            n181 = case shown="False" w483 {
              tunnel: [string[] ["iti mode"] _] -> w482
              frame False {
              }
              frame True {
              }
            }
          }
          frame "mmHelpManual" {
            n182 = call "CFTS-Open Help Topic.vi"("Topic Keyword"="ABR/CAP") -> ()  [unwired: 14 in, 1 out]
          }
        }
      }
      event "CLICK I-O", "TONE I-O": Shortcut Menu Activation? {
        n183 = event-data() -> ()  [unwired: 1 in, 1 out]
        n184 = Unbundle By Name(w497) -> ("Neural"=w496:dbl[][])
        n185 = Empty Array?(array=w496) -> (empty?=w495:bool)
        n186 = event-data("Discard?"=w495) -> ()  [unwired: 1 in, 1 out]
      }
      event "CLICK I-O", "TONE I-O": Shortcut Menu Selection (User) {
        n187 = event-data() -> ()  [unwired: 1 in, 1 out]
        n188 = call "ABR-Estimate Threshold (wrapper).vi"("Analysis (in)"=w504) -> ("Work"=w499:T34, "Analysis (out)"=w503:T14)  [unwired: 12 in, 1 out]
        n189 = call "ABR3-Show Threshold Estimation Work.vi"("work"=w499) -> ()  [unwired: 15 in]
      }
      event "RETURN": Value Change {
        n190 = event-data() -> ()  [unwired: 1 in, 1 out]
      }
      event "START": Value Change {
        n191 = event-data() -> ()  [unwired: 1 in, 1 out]
      }
      event "STOP": Value Change {
        n192 = event-data() -> ()  [unwired: 1 in, 1 out]
        n193 = property on="STOP" class="Bool"("DisabledEnum"=T31."Disabled and Grayed Out" ("Disabled")) -> ()  [unwired: 2 in, 2 out]
      }
      event "result": Value Change {
        w539 = TRUE
        n194 = event-data() -> ("NewVal.error"=w530:errorcluster, "NewVal.aborted"=w537:bool, "NewVal.path"=w525:path)  [unwired: 1 in]
        n195 = property on="RETURN" class="Bool"("Visible"=w539) -> ()  [unwired: 2 in, 2 out]
        n196 = property on="START" class="Bool"("Visible"=w539) -> ()  [unwired: 2 in, 2 out]
        n197 = call "Error Handler.vi"("error in (no error)"=w530) -> ("error?"=w538:bool)  [unwired: 12 in, 2 out]
        n198 = call <vilib>:"Get File Extension.vi"("file"=w525) -> ("filename without extension"=w532:string)  [unwired: 6 in, 4 out]
        n199 = Unbundle By Name(w530) -> ("status"=w529:bool, "code"=w528:i32)
        n200 = Or(x=w538, y=w537) -> (x .or. y?=w536:bool)
        n201 = case shown="True" w536 {
          tunnel: [_ w550] -> w535
          tunnel: w532 -> [_ w547]
          tunnel: w529 -> [_ w546]
          tunnel: w528 -> [_ w545]
          frame False {
            n202 = call "Logger-Log Info.vi"("Message"="Finished" ("message")) -> ()  [unwired: 14 in, 1 out]
          }
          frame True {
            n203 = case shown="False" w546 {
              tunnel: w545 -> [_ w554]
              frame False {
                n204 = call "Logger-Log Info.vi"("Message"="Aborted") -> ()  [unwired: 14 in, 1 out]
              }
              frame True {
                n205 = Format Into String(format string="Error: %d", w554) -> (resulting string=w552:string)  [unwired: 2 in, 1 out]
                n206 = call "Logger-Log Error.vi"("Message"=w552) -> ()  [unwired: 14 in, 1 out]
              }
            }
            n207 = Format Into String(format string="dispose:%s", w547) -> (resulting string=w548:string)  [unwired: 2 in, 1 out]
            n208 = Build Array(w548) -> (w550:string[])
          }
        }
        n209 = Build Array (concatenate)("plot thresh", w535) -> (w533:string[])
        n210 = Bundle By Name(cluster=w540, "running"=FALSE, "path"=w525) -> (w527:cluster{"running":bool, "path":path})
      }
      event Value Change {
        n211 = event-data() -> ("NewVal"=w555:T19)  [unwired: 1 in]
        n212 = Bundle By Name(cluster=w562, "Normalize"=w555) -> (w556:T21)
      }
      event "NOTES": Value Change {
        n213 = event-data() -> ("NewVal"=w576:string)  [unwired: 1 in]
        n214 = Unbundle By Name(w566) -> ("path"=w565:path, "running"=w564:bool)
        n215 = Not(x=w564) -> (.not. x?=w570:bool)
        n216 = Empty String/Path?(string/path=w565) -> (empty?=w571:bool)
        n217 = Not(x=w571) -> (.not. x?=w569:bool)
        n218 = And(x=w569, y=w570) -> (x .and. y?=w568:bool)
        n219 = case shown="True" w568 {
          tunnel: w565 -> [_ w582]
          tunnel: w576 -> [_ w581]
          tunnel: "Add notes to data file?" ("message") -> [_ w580]
          tunnel: "STANDARD ABR" -> [_ w577]
          frame False {
          }
          frame True {
            n220 = Two Button Dialog(message=w580) -> (T button?=w579:bool)  [unwired: 2 in]
            n221 = case shown="True" w579 {
              tunnel: w582 -> [_ w586]
              tunnel: w581 -> [_ w585]
              tunnel: "Notes" -> [_ w584]
              tunnel: w577 -> [_ w583]
              frame False {
              }
              frame True {
                n222 = call-poly "Config-Write Key.vi"("configuration file path"=w586, "section"=w583, "key"=w584, "value"=w585) -> ()  [unwired: 9 in, 3 out]
              }
            }
          }
        }
      }
      event "Stimulus": Value Change {
        n223 = event-data() -> ()  [unwired: 1 in, 1 out]
      }
      event "CAP or ABR": Value Change {
        n224 = event-data() -> ()  [unwired: 1 in, 1 out]
        n225 = Bundle By Name(cluster=w599, "Response.CAP or ABR"="CAP or ABR") -> (w598:T21)
      }
      event "Response": Value Change {
        n226 = event-data() -> ()  [unwired: 1 in, 1 out]
      }
      event Value Change {
        n227 = event-data() -> ("NewVal"=w609:T14)  [unwired: 1 in]
      }
    }
  }
